vi "read channel page caen.vi"(0 "VISA in":refnum<visa-resource-name>, 5 "Crate":i32, 7 "page":i32, 11 "error in":errorcluster) -> (4 "VISA out":refnum<visa-resource-name>, 6 "Array":T1[](array[typedef]) {"Vfile (V)" format="%.1f V"; "Vswmax (V)" format="%#_g V"; "Iset (A)" format="%.2pA"; "Imon (A)" format="%.2pA"; "Vset (V)" format="%#_g V"; "Vmon (V)" format="%.1f V"}, 8 "New Channels":T1[](array[typedef]) {"Vfile (V)" format="%.1f V"; "Vswmax (V)" format="%#_g V"; "Iset (A)" format="%.2pA"; "Imon (A)" format="%.2pA"; "Vset (V)" format="%#_g V"; "Vmon (V)" format="%.1f V"}, 10 "Start Index in ACTIVE":i32, 15 "error out":errorcluster)   [LabVIEW 2018]
uses:
  channel_cluster.ctl
  set location.ctl
  channel.ctl
  CAEN globals.vi
  <userlib>/_OpenG.lib/array/array.llb/Filter 1D Array with Scalar (I32)__ogtk.vi
  <vilib>/Utility/file.llb/Write Delimited Spreadsheet (string).vi
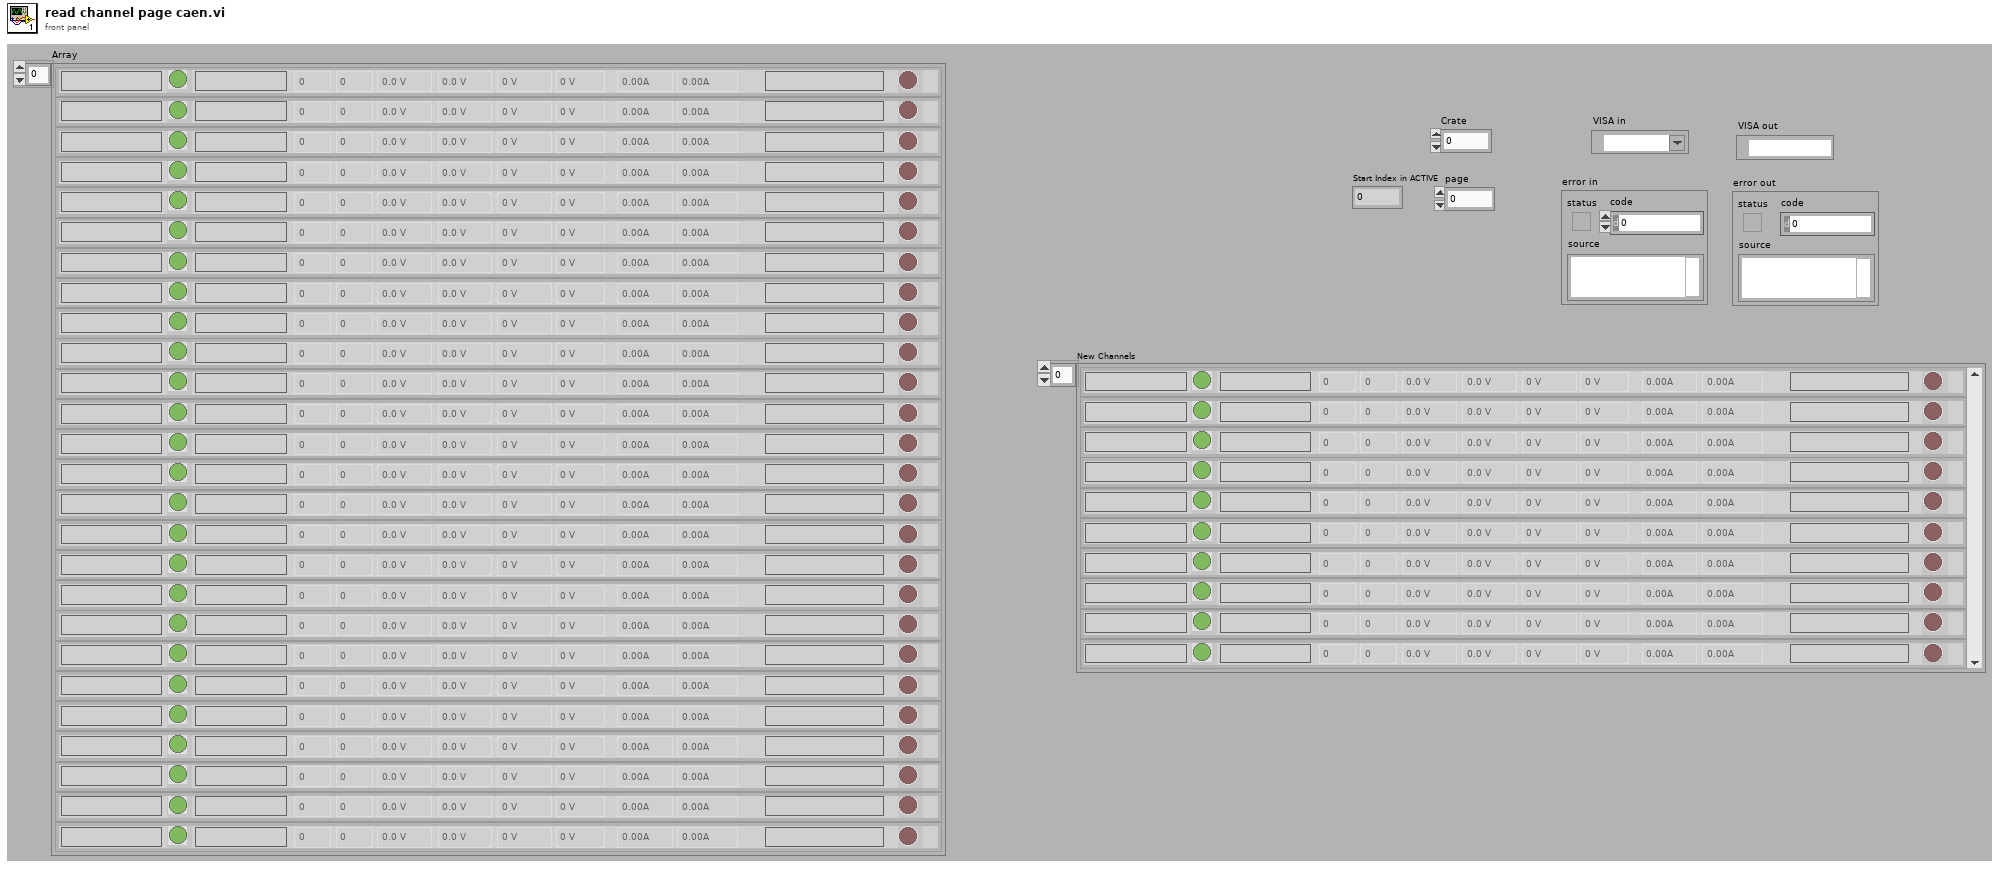
[diagram p1: front panel]
types:
  T1 = typedef "channel_cluster.ctl" = cluster{"Channel Name":string, "Crate":i32, "Card Type":string, "Card":i32, "Channel":i32, "Status Icon":picture, "Vmon (V)":dbl, "Vset (V)":dbl, "Imon (A)":dbl, "Iset (A)":dbl, "Timestamp":string, "ON/OFF":bool, "Status":string, "Vswmax (V)":dbl, "Flag":bool, "Vfile (V)":dbl, "Error Logged":bool[], "enable_file":bool}
  T2 = typedef "channel.ctl" = cluster{" Card.Channel":dbl, "Crate":i32}
  T3 = typedef "set location.ctl" = cluster{"set index":i32, "set Screen":string, "set subpage":i32, "set column":i32, "Group":string, "Crate":i32}
  T4 = typedef "location cluster.ctl" = cluster{"Column":i32, "Card Type":string, "Channel":i32, "Card":i32, "Default response":string, "Entering":string, "Entering state":bool, "subpage":i32, "page":i32, "Crate":i32, "Screen":string, "Group":string, "Global HV Enable":bool, "Vsel_buffer":bool, "Vdisp_buffer":bool}
  T5 = typedef "crate.ctl" = cluster{"CAENet Address":i32, "Crate Model":string, "Firmware Version":string, "Crate Map":T6[], "Total Channels":i32}
  T6 = typedef "card.ctl" = cluster{"Slot Number":i32, "Card Model":string, "Num Channels":i32, "Polarity":string, "Vmax":dbl, "Imax":dbl, "Revision":string}
  T7 = cluster{"Group Name":string, "Channels in Group":T2[]}[]
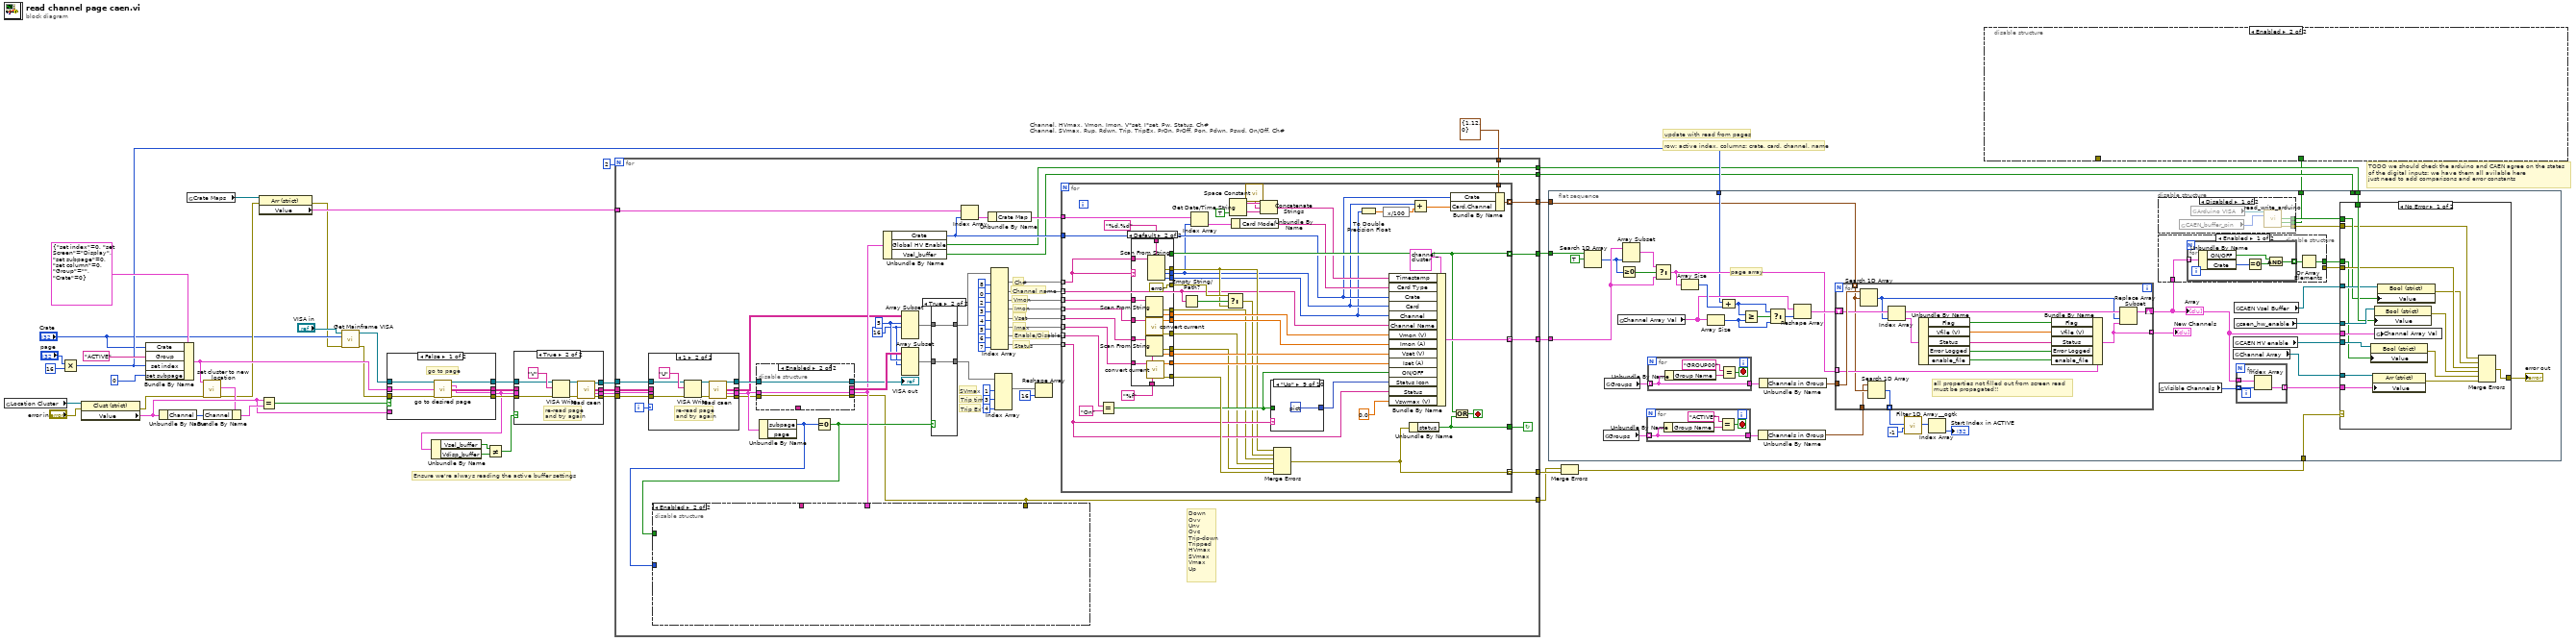
[diagram p0: block diagram]
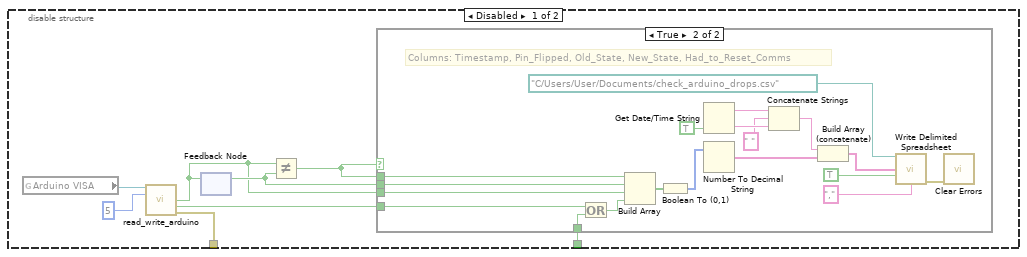
[diagram p2: hidden frame]
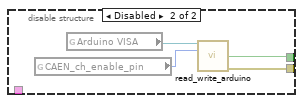
[diagram p6: hidden frame]
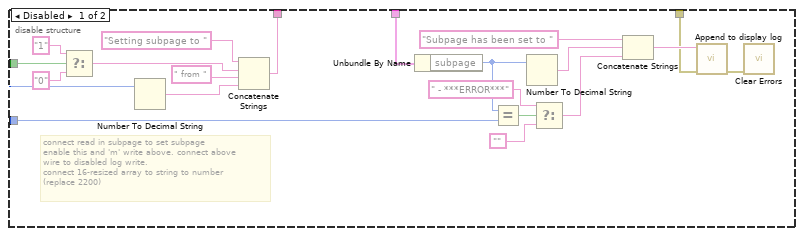
[diagram p9: hidden frame]
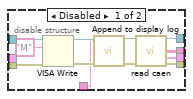
[diagram p10: hidden frame]
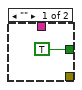
[diagram p12: hidden frame]
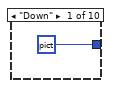
[diagram p13: hidden frame]
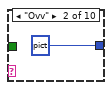
[diagram p14: hidden frame]
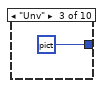
[diagram p15: hidden frame]
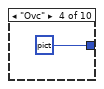
[diagram p16: hidden frame]
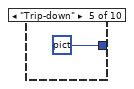
[diagram p17: hidden frame]
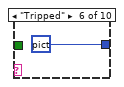
[diagram p18: hidden frame]
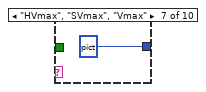
[diagram p19: hidden frame]
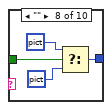
[diagram p20: hidden frame]
diagram:
  # "Ensure we're always reading the active buffer settings"
  # "TODO we should check the arduino and CAEN agree on the states\nof the digital inputs: we have them all avilable here\njust need to add comparisons and error constants"
  # "row: active index, columns: crate, card, channel, name"
  # "update with read from pages"
  # "Channel, HVmax, Vmon, Imon, V*set, I*set, Pw, Status, Ch#\nChannel, SVmax, Rup, Rdwn, Trip, TripEx, PrOn, PrOff, Pon, Pdwn, Pswd, On/Off, Ch#"
  n1 = global read "CAEN globals.vi" "Location Cluster"() -> (w40:refnum<vi>)
  n2 = Multiply(x="page", y=16) -> (x*y=w21:i32)
  n3 = property class="Clust (strict)"(reference=w40, error in="error in") -> (error out=w33:errorcluster, "Value"=w36:T4)  [unwired: 1 out]
  n4 = Bundle By Name(cluster=T3 {"set index"=0, "set Screen"="Display", "set subpage"=0, "set column"=0, "Group"="", "Crate"=0} ("Set Cluster"), "Crate"="Crate", "Group"="ACTIVE", "set index"=w21, "set subpage"=0) -> (w38:T3)
  n5 = Unbundle By Name(w36) -> ("Channel"=w32:i32)
  n6 = global read "CAEN globals.vi" "Crate Maps"() -> (w27:refnum<vi>)
  n7 = call "set cluster to new location.vi"("error in"=w33, "Set Cluster"=w38) -> ("error out"=w26:errorcluster, "Location Cluster out"=w31:T4)  [unwired: 6 in, 2 out]
  n8 = Bundle By Name(cluster=w31, "Channel"=w32) -> (w37:T4)
  n9 = property class="Arr (strict)"(reference=w27, error in=w26) -> (error out=w16:errorcluster, "Value"=w25:T5[])  [unwired: 1 out]
  n10 = Equal?(x=w36, y=w37) -> (x = y?=w35:bool)
  n11 = call "Get Mainframe VISA.vi"("Error In"=w16, "Crate"="Crate", "VISA In"="VISA in") -> ("Error Out"=w15:errorcluster, "VISA out"=w18:refnum<visa-resource-name>)  [unwired: 6 in, 1 out]
  n12 = case shown="False" w35 {
    tunnel: [w52 w54] -> w6
    tunnel: [w51 w56] -> w12
    tunnel: [w50 w55] -> w7
    tunnel: w18 -> [w49 w64]
    tunnel: w15 -> [w48 w63]
    tunnel: w38 -> [w47 _]
    tunnel: w36 -> [_ w62]
    tunnel: [w46 w53] -> w5
    frame False {
      # "go to page"
      n13 = call "go to desired page.vi"("VISA in"=w49, "Set Cluster"=w47, "error in"=w48) -> ("VISA out"=w50:refnum<visa-resource-name>, "Location Cluster out"=w46:T4, "Display array"=w52:string[][], "error out"=w51:errorcluster)  [unwired: 9 in]
    }
    frame True {
      # "just refresh"
      # "already there"
      n14 = call "handle entering.vi"("VISA in"=w64, "Current location"=w62, "error in"=w63) -> ("VISA out"=w61:refnum<visa-resource-name>, "error out"=w60:errorcluster)  [unwired: 14 in, 1 out]
      n15 = VISA Write(VISA resource name=w61, write buffer="U", error in (no error)=w60) -> (VISA resource name out=w58:refnum<visa-resource-name>, error out=w57:errorcluster)  [unwired: 1 out]
      n16 = call "read caen.vi"("VISA in"=w58, "error in"=w57) -> ("VISA out"=w55:refnum<visa-resource-name>, "Display array"=w54:string[][], "Location Cluster"=w53:T4, "error out"=w56:errorcluster)  [unwired: 8 in, 2 out]
    }
  }
  n17 = Unbundle By Name(w5) -> ("Vsel_buffer"=w4:bool, "Vdisp_buffer"=w3:bool)
  n18 = Not Equal?(x=w4, y=w3) -> (x != y?=w2:bool)
  n19 = case shown="True" w2 {
    tunnel: w12 -> [w67 w74]
    tunnel: [w67 w73] -> w11
    tunnel: [w65 w72] -> w10
    tunnel: [w66 w71] -> w9
    tunnel: [w68 w70] -> w8
    tunnel: w7 -> [w68 w69]
    tunnel: w6 -> [w66 _]
    tunnel: w5 -> [w65 _]
    frame False {
    }
    frame True {
      # "re-read page\nand try again"
      n20 = VISA Write(VISA resource name=w69, write buffer="V", error in (no error)=w74) -> (VISA resource name out=w76:refnum<visa-resource-name>, error out=w77:errorcluster)  [unwired: 1 out]
      n21 = call "read caen.vi"("VISA in"=w76, "error in"=w77) -> ("VISA out"=w70:refnum<visa-resource-name>, "Display array"=w71:string[][], "Location Cluster"=w72:T4, "error out"=w73:errorcluster)  [unwired: 8 in, 2 out]
    }
  }
  n22 = for {
    N: 2 -> [_]
    tunnel: w8 -> [w98]
    tunnel: [w110] -> w45
    tunnel: [w109] -> w42
    tunnel: [w108] -> w41
    tunnel: w10 -> [w93]
    tunnel: w9 -> [w92]
    tunnel: w11 -> [w94]
    tunnel: [w86] -> w30
    tunnel: w25 -> [w83]
    tunnel: T2 {" Card.Channel"=1.12, "Crate"=0} ("Cluster") -> [w79]
    tunnel: [w82] -> w23
    tunnel: [w80] -> w20
    tunnel: [w78] -> w13
    i -> [w96]
    stop <- w87 continue-if-true
    w129 = 16 ("index")
    w130 = 5 ("index")
    # "Ch#"
    # "Down\nOvv\nUnv\nOvc\nTrip-down\nTripped\nHVmax\nSVmax\nVmax\nUp"
    # "Channel name"
    # "Trip Ex??"
    # "Trip time"
    # "SVmax"
    # "Status"
    # "Enable/Disable"
    # "Imax"
    # "Vset"
    # "Imon"
    # "Vmon"
    n23 = case shown="1" w96 {
      tunnel: [w132 w139] -> w89
      tunnel: [w134 w141] -> w90
      tunnel: [w135 w140] -> w97
      tunnel: w98 -> [w135 w137]
      tunnel: [w133 w138] -> w91
      tunnel: w94 -> [w134 w136]
      tunnel: w93 -> [w133 _]
      tunnel: w92 -> [w132 _]
      frame 0, Default {
      }
      frame 1 {
        # "re-read page\nand try again"
        n24 = VISA Write(VISA resource name=w137, write buffer="U", error in (no error)=w136) -> (VISA resource name out=w143:refnum<visa-resource-name>, error out=w142:errorcluster)  [unwired: 1 out]
        n25 = call "read caen.vi"("VISA in"=w143, "error in"=w142) -> ("VISA out"=w140:refnum<visa-resource-name>, "Display array"=w139:string[][], "Location Cluster"=w138:T4, "error out"=w141:errorcluster)  [unwired: 8 in, 2 out]
      }
    }
    n26 = disable-structure shown="Enabled" {
      disable-tunnel: [w175 _] -> w131
      disable-tunnel: [w174 w178] -> w128
      disable-tunnel: w90 -> [w173 w177]
      disable-tunnel: w97 -> [w172 w178]
      disable-tunnel: _ -> [w167 _]
      disable-tunnel: [w166 w177] -> w86
      disable-tunnel: [w165 w176] -> w99
      disable-tunnel: w91 -> [_ w176]
      frame Disabled {
        n27 = VISA Write(VISA resource name=w172, write buffer="M", error in (no error)=w173) -> (VISA resource name out=w171:refnum<visa-resource-name>, error out=w169:errorcluster)  [unwired: 1 out]
        n28 = call "Append to display log.vi"("error in"=w169, "string"=w167) -> ("error out"=w168:errorcluster)  [unwired: 9 in]
        n29 = call "read caen.vi"("VISA in"=w171, "error in"=w168) -> ("VISA out"=w174:refnum<visa-resource-name>, "Display array"=w175:string[][], "Location Cluster"=w165:T4, "error out"=w166:errorcluster)  [unwired: 8 in, 2 out]
      }
      frame Enabled {
      }
    }
    "VISA out" <- w128
    n30 = Unbundle By Name(w91) -> ("subpage"=w88:i32)  [unwired: 1 out]
    n31 = Equal To 0?(x=w88) -> (x = 0?=w95:bool)
    n32 = disable-structure shown="Enabled" {
      disable-tunnel: [w164 _] -> _
      disable-tunnel: w95 -> [w163 _]
      disable-tunnel: w88 -> [w153 _]
      disable-tunnel: w86 -> [w152 _]
      disable-tunnel: w99 -> [w151 _]
      frame Disabled {
        # "connect read in subpage to set subpage\nenable this and 'm' write above. connect above\nwire to disabled log write.\nconnect 16-resized array to string to number\n(replace 2200)"
        n33 = Select(t="1" ("string"), s=w163, f="0" ("string")) -> (s? t:f=w146:string)
        n34 = Number To Decimal String(number=w153) -> (decimal integer string=w145:string)  [unwired: 1 in]
        n35 = Concatenate Strings("Setting subpage to " ("string"), w146, " from " ("string"), w145) -> (w164:string)
        n36 = Unbundle By Name(w151) -> ("subpage"=w154:i32)
        n37 = Equal?(x=w154, y=w153) -> (x = y?=w155:bool)
        n38 = Number To Decimal String(number=w154) -> (decimal integer string=w161:string)  [unwired: 1 in]
        n39 = Select(t=" - ***ERROR***" ("string"), s=w155, f="") -> (s? t:f=w158:string)
        n40 = Concatenate Strings("Subpage has been set to " ("string"), w161, w158) -> (w157:string)
        n41 = call "Append to display log.vi"("error in"=w152, "string"=w157) -> ("error out"=w156:errorcluster)  [unwired: 9 in]
        n42 = call <vilib>:"Clear Errors.vi"("error in (no error)"=w156) -> ()  [unwired: 5 in, 2 out]
      }
      frame Enabled {
      }
    }
    n43 = Unbundle By Name(w99) -> ("Crate"=w81:i32, "Global HV Enable"=w80:bool, "Vsel_buffer"=w78:bool)
    n44 = Array Subset(array=w89, index (row)=w130, length (row)=w129) -> (w107:string[][])  [unwired: 2 in]
    n45 = Array Subset(array=w131, index (row)=w130, length (row)=w129) -> (w106:string[][])  [unwired: 2 in]
    n46 = case shown="True" w95 {
      tunnel: w107 -> [w180 w182]
      tunnel: w106 -> [w179 w181]
      tunnel: [w179 w182] -> w105
      tunnel: [w180 w181] -> w104
      frame False {
      }
      frame True {
      }
    }
    n47 = Index Array(array=w83, index=w81) -> (element=w85:T5)
    n48 = Unbundle By Name(w85) -> ("Crate Map"=w84:T6[])
    n49 = Index Array(array=w105, index (col) #1=8 ("disabled index (col)"), index (col) #2=0 ("disabled index (col)"), index (col) #3=2 ("disabled index (col)"), index (col) #4=3 ("disabled index (col)"), index (col) #5=4 ("disabled index (col)"), index (col) #6=5 ("disabled index (col)"), index (col) #7=6 ("disabled index (col)"), index (col) #8=7 ("disabled index (col)")) -> (element #1=w100:string[], element #2=w127:string[], element #3=w126:string[], element #4=w125:string[], element #5=w124:string[], element #6=w123:string[], element #7=w122:string[], element #8=w121:string[])  [unwired: 8 in]
    n50 = Index Array(array=w104, index (col) #1=1 ("disabled index (col)"), index (col) #2=3 ("disabled index (col)"), index (col) #3=4 ("disabled index (col)")) -> (element #1=w103:string[])  [unwired: 3 in, 2 out]
    n51 = Reshape Array(w103, 16 ("dimension size")) -> ()  [unwired: 1 out]
    n52 = for {
      tunnel: w127 -> [w186] mode=indexing
      tunnel: w126 -> [w208] mode=indexing
      tunnel: w125 -> [w220] mode=indexing
      tunnel: w124 -> [w207] mode=indexing
      tunnel: w123 -> [w229] mode=indexing
      tunnel: w122 -> [w221] mode=indexing
      tunnel: w121 -> [w219] mode=indexing
      tunnel: [w216] -> w110 mode=indexing
      tunnel: [w223] -> w108 mode=indexing
      tunnel: [w204] -> w109 mode=indexing
      tunnel: w100 -> [w205] mode=indexing
      tunnel: w81 -> [w185]
      tunnel: [w200] -> w87
      tunnel: w84 -> [w198]
      tunnel: w79 -> [w189]
      tunnel: [w187] -> w82 mode=indexing
      stop <- w215 stop-if-true
      n53 = Equal?(x=w221, y="On") -> (x = y?=w218:bool)
      n54 = case shown="Default" w205 {
        tunnel: w220 -> [_ w250]
        tunnel: [_ w249] -> w230
        tunnel: w229 -> [_ w248]
        tunnel: [_ w247] -> w212
        tunnel: [_ w246] -> w201
        tunnel: [_ w245] -> w228
        tunnel: [_ w244] -> w210
        tunnel: [_ w243] -> w209
        tunnel: w208 -> [_ w242]
        tunnel: w207 -> [_ w241]
        tunnel: [_ w240] -> w206
        tunnel: [_ w239] -> w202
        tunnel: w205 -> [_ w238]
        tunnel: [_ w237] -> w191
        tunnel: "%d.%d" ("y") -> [_ w236]
        tunnel: [TRUE ("want seconds? (F)") _] -> w204
        tunnel: [_ w235] -> w184
        tunnel: [_ w234] -> w183
        tunnel: "%f" ("y") -> [_ w233]
        tunnel: [_ errorcluster {"status"=TRUE, "code"=0, "source"="Name read error"} ("error out")] -> w192
        frame "" {
        }
        frame Default {
          n55 = Scan From String(format string=w233, input string=w242) -> (error out=w243:errorcluster, output 1=w244:dbl)  [unwired: 3 in, 2 out]
          n56 = call "convert current.vi"("input string"=w250) -> ("error IO"=w246:errorcluster, "Numeric"=w249:dbl)  [unwired: 3 in, 2 out]
          n57 = Scan From String(format string=w233, input string=w241) -> (error out=w239:errorcluster, output 1=w240:dbl)  [unwired: 3 in, 2 out]
          n58 = call "convert current.vi"("input string"=w248) -> ("error IO"=w245:errorcluster, "Numeric"=w247:dbl)  [unwired: 3 in, 2 out]
          n59 = Scan From String(format string=w236, input string=w238) -> (error out=w237:errorcluster, output 1=w235:i32, output 2=w234:i32)  [unwired: 4 in, 2 out]
        }
      }
      n60 = Empty String/Path?(string/path=w186) -> (empty?=w194:bool)
      n61 = Index Array(array=w198, index=w184) -> (element=w197:T6)
      n62 = Select(t=w192, s=w194, f=w191) -> (s? t:f=w193:errorcluster)
      n63 = Get Date/Time String(want seconds? (F)=TRUE) -> (date string=w227:string, time string=w226:string)  [unwired: 2 in]
      n64 = Unbundle By Name(w197) -> ("Card Model"=w195:string)
      n65 = call <vilib>:"Space Constant.vi"() -> ("String"=w225:string)
      n66 = Concatenate Strings(w227, w225, w226) -> (w196:string)
      n67 = case shown="\"Up\"" w219 {
        tunnel: w218 -> [_ _ _ _ _ _ _ w258 _ _]
        tunnel: [picture bytes[830] ("Status Icon") picture bytes[930] ("Status Icon 2") picture bytes[930] ("Status Icon 2") picture bytes[830] ("Status Icon 2") picture bytes[830] ("Status Icon 2") picture bytes[780] ("Status Icon 2") picture bytes[930] ("Status Icon 2") w261 picture bytes[830] ("Status Icon 2") picture data[5B] ("Status Icon 2")] -> w217
        frame "Down" {
        }
        frame "Ovv" {
        }
        frame "Unv" {
        }
        frame "Ovc" {
        }
        frame "Trip-down" {
        }
        frame "Tripped" {
        }
        frame "HVmax", "SVmax", "Vmax" {
        }
        frame "" {
          n68 = Select(t=picture bytes[830] ("Status Icon 2"), s=w258, f=picture bytes[830] ("new picture 2")) -> (s? t:f=w261:picture)
        }
        frame "Up" {
        }
        frame Default {
        }
      }
      n69 = Merge Errors(w191, w193, w209, w201, w202, w228) -> (w216:errorcluster)
      n70 = To Double Precision Float(number=w183) -> (double precision float=w213:dbl)
      n71 = expression code="x/100"(w213) -> (w214:dbl)
      n72 = Bundle By Name(cluster=T1 {"Channel Name"="", "Crate"=0, "Card Type"="", "Card"=0, "Channel"=0, "Status Icon"=bytes[0], "Vmon (V)"=0.0, "Vset (V)"=0.0, "Imon (A)"=0.0, "Iset (A)"=0.0, "Timestamp"="", "ON/OFF"=FALSE, "Status"="", "Vswmax (V)"=0.0, "Flag"=FALSE, "Vfile (V)"=0.0, "Error Logged"=[], "enable_file"=FALSE} ("Channel cluster"), "Timestamp"=w196, "Card Type"=w195, "Crate"=w185, "Card"=w184, "Channel"=w183, "Channel Name"=w186, "Vmon (V)"=w210, "Imon (A)"=w230, "Vset (V)"=w206, "Iset (A)"=w212, "ON/OFF"=w218, "Status Icon"=w217, "Status"=w219, "Vswmax (V)"=0.0 ("number")) -> (w223:T1)
      n73 = Unbundle By Name(w216) -> ("status"=w200:bool)
      n74 = Add(x=w184, y=w214) -> (x+y=w188:dbl)
      n75 = Bundle By Name(cluster=w189, "Crate"=w185, "Card.Channel"=w188) -> (w187:T2)
      n76 = Or(x=w204, y=w200) -> (x .or. y?=w215:bool)
    }
  }
  n77 = flat-sequence {
    tunnel: w42 -> [w300]
    tunnel: w41 -> [w296]
    tunnel: w23 -> [w277]
    tunnel: w22 -> [w285]
    tunnel: w21 -> [w284]
    tunnel: w20 -> [w281]
    tunnel: w13 -> [_]
    tunnel: [w264] -> w1
    frame #0 {
      # "page array"
      n78 = Search 1D Array(1D array=w300, element=TRUE) -> (index of element=w295:i32)  [unwired: 1 in]
      n79 = global read "CAEN globals.vi" "Groups"() -> (w279:T7)
      n80 = global read "CAEN globals.vi" "Groups"() -> (w288:T7)
      n81 = global read "CAEN globals.vi" "Channel Array Val"() -> (w289:T1[])
      n82 = Greater Or Equal To 0?(x=w295) -> (x >= 0?=w298:bool)
      n83 = Array Subset(array=w296, length=w295) -> (w297:T1[])  [unwired: 1 in]
      n84 = for {
        tunnel: w279 -> [w324] mode=indexing
        tunnel: [w324] -> w278
        stop <- w323 stop-if-true
        n85 = Unbundle By Name(w324) -> ("Group Name"=w326:string)
        n86 = Equal?(x="ACTIVE" ("Group Name"), y=w326) -> (x = y?=w323:bool)
      }
      n87 = for {
        tunnel: w288 -> [w328] mode=indexing
        tunnel: [w328] -> w287
        stop <- w327 stop-if-true
        n88 = Unbundle By Name(w328) -> ("Group Name"=w330:string)
        n89 = Equal?(x="GROUP00" ("Group Name"), y=w330) -> (x = y?=w327:bool)
      }
      n90 = Select(t=w297, s=w298, f=w296) -> (s? t:f=w294:T1[])
      n91 = Array Size(array=w294) -> (size(s)=w293:i32)
      n92 = Array Size(array=w289) -> (size(s)=w304:i32)
      n93 = Compound Arithmetic op=ADD(w284, w293) -> (w301:i32)
      n94 = Greater Or Equal?(x=w301, y=w304) -> (x >= y?=w305:bool)
      n95 = Unbundle By Name(w278) -> ("Channels in Group"=w276:T2[])
      n96 = Unbundle By Name(w287) -> ("Channels in Group"=w286:T2[])
      n97 = Select(t=w301, s=w305, f=w304) -> (s? t:f=w303:i32)
      n98 = Reshape Array(w289, w303) -> (w302:T1[])
      n99 = for {
        tunnel: w294 -> [w338] mode=indexing
        shift-right: [w345] -> w270
        shift-left: w302 -> [w343]
        tunnel: w286 -> [w344]
        tunnel: w277 -> [w333] mode=indexing
        tunnel: [w336] -> w280 mode=indexing
        tunnel: w276 -> [w332]
        tunnel: [w331] -> w275 mode=indexing
        # "all properties not filled out from screen read\nmust be propagated!!"
        n100 = Search 1D Array(1D array=w344, element=w333) -> (index of element=w342:i32)  [unwired: 1 in]
        n101 = Search 1D Array(1D array=w332, element=w333) -> (index of element=w331:i32)  [unwired: 1 in]
        n102 = Index Array(array=w343, index=w342) -> (element=w341:T1)
        n103 = Unbundle By Name(w341) -> ("Flag"=w340:bool, "Vfile (V)"=w339:dbl, "Status"=w337:string, "Error Logged"=w335:bool[], "enable_file"=w334:bool)
        n104 = Bundle By Name(cluster=w338, "Flag"=w340, "Vfile (V)"=w339, "Status"=w337, "Error Logged"=w335, "enable_file"=w334) -> (w336:T1)
        n105 = Replace Array Subset(array=w343, new element=w336, index=w342) -> (w345:T1[])
      }
      "Array" <- w270
      "New Channels" <- w280
      n106 = call-poly <userlib>:"Filter 1D Array__ogtk.vi"("items to filter"=-1 ("Numeric"), "array"=w275) -> ("filtered array"=w273:i32[])  [unwired: 4 in, 1 out]
      n107 = Index Array(array=w273) -> (element=→"Start Index in ACTIVE":i32)  [unwired: 1 in]
      n108 = disable-structure shown="Disabled" {
        disable-tunnel: [w308 _] -> w266
        disable-tunnel: [w307 _] -> w265
        disable-tunnel: [w306 _] -> w264
        frame Disabled {
          n109 = global read "CAEN globals.vi" "CAEN_buffer_pin"() -> (w310:u8)
          n110 = global read "CAEN globals.vi" "Arduino VISA"() -> (w309:refnum<visa-resource-name>)
          n111 = call "read_write_arduino.vi"("VISA in"=w309, "Pin Num"=w310) -> ("State"=w308:bool, "Comms Reset"=w306:bool, "error out"=w307:errorcluster)  [unwired: 10 in, 1 out]
        }
        frame Enabled {
        }
      }
      n112 = disable-structure shown="Enabled" {
        disable-tunnel: w270 -> [w313 _]
        disable-tunnel: [w311 w319] -> w269
        disable-tunnel: [_ w320] -> w268
        frame Enabled {
          n113 = for {
            tunnel: w313 -> [w318] mode=indexing
            tunnel: [w314] -> w312 mode=indexing
            n114 = Unbundle By Name(w318) -> ("ON/OFF"=w315:bool, "Crate"=w317:i32)
            n115 = Equal To 0?(x=w317) -> (x = 0?=w316:bool)
            n116 = And(x=w315, y=w316) -> (x .and. y?=w314:bool)
          }
          n117 = Or Array Elements(Boolean array=w312) -> (logical OR=w311:bool)
        }
        frame Disabled {
          n118 = global read "CAEN globals.vi" "CAEN_ch_enable_pin"() -> (w321:u8)
          n119 = global read "CAEN globals.vi" "Arduino VISA"() -> (w322:refnum<visa-resource-name>)
          n120 = call "read_write_arduino.vi"("VISA in"=w322, "Pin Num"=w321) -> ("State"=w319:bool, "error out"=w320:errorcluster)  [unwired: 10 in, 2 out]
        }
      }
      n121 = global read "CAEN globals.vi" "Visible Channels"() -> (w291:i32[])
      n122 = global read "CAEN globals.vi" "CAEN HV enable"() -> (w282:refnum<vi>)
      n123 = global read "CAEN globals.vi" "Channel Array"() -> (w292:refnum<vi>)
      n124 = global read "CAEN globals.vi" "CAEN Vsel Buffer"() -> (w267:refnum<vi>)
      n125 = global read "CAEN globals.vi" "caen_hw_enable"() -> (w271:refnum<vi>)
      n126 = for {
        tunnel: w291 -> [w364] mode=indexing
        tunnel: w270 -> [w365]
        tunnel: [w363] -> w290 mode=indexing
        n127 = Index Array(array=w365, index=w364) -> (element=w363:T1)
      }
      n128 = case shown="No Error" w285 {
        selector: w285 -> [_ w362]
        tunnel: w292 -> [w361 _]
        tunnel: w270 -> [w360 _]
        tunnel: w290 -> [w359 _]
        tunnel: [w356 w362] -> w283
        tunnel: w282 -> [w355 _]
        tunnel: w281 -> [w352 _]
        tunnel: w271 -> [w354 _]
        tunnel: w269 -> [w348 _]
        tunnel: w268 -> [w351 _]
        tunnel: w267 -> [w349 _]
        tunnel: w266 -> [w347 _]
        tunnel: w265 -> [w346 _]
        frame No Error {
          n129 = property class="Bool (strict)"(reference=w355, "Value"=w348) -> (error out=w357:errorcluster)  [unwired: 1 in, 1 out]
          n130 = property class="Arr (strict)"(reference=w361, "Value"=w359) -> (error out=w358:errorcluster)  [unwired: 1 in, 1 out]
          n131 = property class="Bool (strict)"(reference=w354, "Value"=w352) -> (error out=w353:errorcluster)  [unwired: 1 in, 1 out]
          n132 = global write "CAEN globals.vi" "Channel Array Val"(w360) -> ()
          n133 = property class="Bool (strict)"(reference=w349, "Value"=w347) -> (error out=w350:errorcluster)  [unwired: 1 in, 1 out]
          n134 = Merge Errors(w346, w350, w351, w353, w357, w358) -> (w356:errorcluster)
        }
        frame Error {
        }
      }
      "error out" <- w283
    }
  }
  n135 = Merge Errors(w30, w45) -> (w22:errorcluster)
  n136 = disable-structure shown="Enabled" {
    disable-tunnel: [w372 _] -> _
    disable-tunnel: w1 -> [w369 _]
    frame Disabled {
      n137 = global read "CAEN globals.vi" "Arduino VISA"() -> (w373:refnum<visa-resource-name>)
      n138 = call "read_write_arduino.vi"("VISA in"=w373, "Pin Num"=u8 5) -> ("State"=w366:bool, "Comms Reset"=w370:bool, "error out"=w372:errorcluster)  [unwired: 10 in, 1 out]
      n139 = feedback #1() -> (w367:bool)  [unwired: 1 in]
      n140 = feedback-in #1(w366) -> ()
      n141 = Not Equal?(x=w366, y=w367) -> (x != y?=w368:bool)
      n142 = case shown="True" w368 {
        tunnel: w370 -> [_ w392]
        tunnel: w369 -> [_ w391]
        tunnel: w368 -> [_ w389]
        tunnel: w367 -> [_ w375]
        tunnel: w366 -> [_ w374]
        frame False {
        }
        frame True {
          # "Columns: Timestamp, Pin_Flipped, Old_State, New_State, Had_to_Reset_Comms"
          n143 = Or(x=w392, y=w391) -> (x .or. y?=w390:bool)
          n144 = Build Array(w389, w375, w374, w390) -> (w388:bool[])
          n145 = Boolean To (0,1)(Boolean=w388) -> (0, 1=w383:i16[])
          n146 = Get Date/Time String(want seconds? (F)=TRUE) -> (date string=w381:string, time string=w380:string)  [unwired: 2 in]
          n147 = Number To Decimal String(number=w383) -> (decimal integer string=w378:string[])  [unwired: 1 in]
          n148 = Concatenate Strings(w381, " " ("delimiter (\\t)"), w380) -> (w377:string)
          n149 = Build Array (concatenate)(w377, w378) -> (w376:string[])
          n150 = call-poly <vilib>:"Write Delimited Spreadsheet.vi"("file path (dialog if empty)"=path "C:/Users/User/Documents/check_arduino_drops.csv", "1D data"=w376, "append to file? (new file:F)"=TRUE, "delimiter (\\t)"="," ("delimiter (\\t)")) -> ("error out"=w384:errorcluster)  [unwired: 10 in, 1 out]
          n151 = call <vilib>:"Clear Errors.vi"("error in (no error)"=w384) -> ()  [unwired: 5 in, 2 out]
        }
      }
    }
    frame Enabled {
    }
  }
